vi "Read Message.vi"(8 "error in (no error)":errorcluster, 9 "timeout (0)":i32, 11 "Master CR in":refnum<class "Master CR.lvclass">) -> (0 "error out":errorcluster, 1 "timed out?":bool, 3 "Master CR out":refnum<class "Master CR.lvclass">)   [LabVIEW 2021, in "Master CR.lvclass"]
uses:
  Master CR.lvclass
  Master CR.lvclass/Master CR.ctl
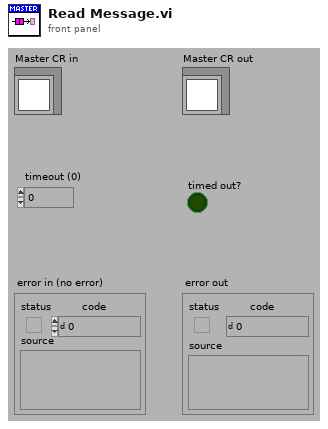
[diagram p1: front panel]
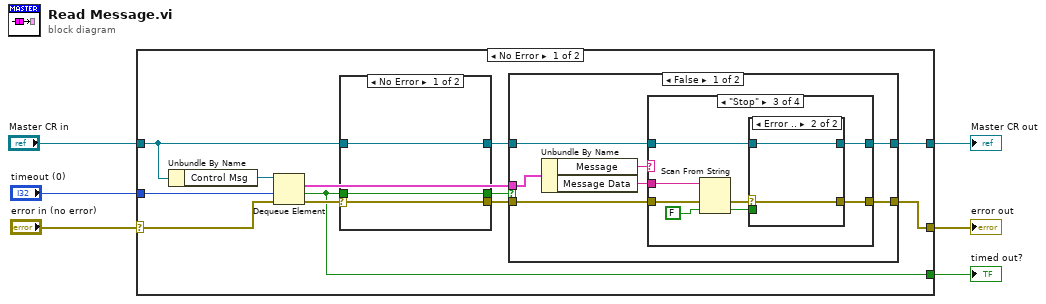
[diagram p0: block diagram]
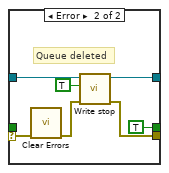
[diagram p2: hidden frame]
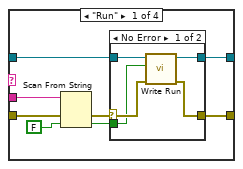
[diagram p3: hidden frame]
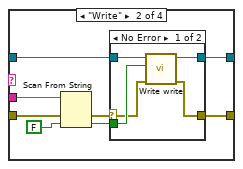
[diagram p5: hidden frame]
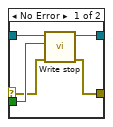
[diagram p7: hidden frame]
diagram:
  n1 = case shown="No Error" "error in (no error)" {
    selector: "error in (no error)" -> [w17 w86]
    tunnel: [w13 w86] -> w6
    tunnel: "timeout (0)" -> [w18 _]
    tunnel: [w14 w85] -> w1
    tunnel: [w10 _] -> w3
    tunnel: "Master CR in" -> [w8 w85]
    frame No Error {
      n2 = Unbundle By Name(w8) -> ("Control Msg"=w16:refnum<queue>)
      n3 = Dequeue Element(queue=w16, timeout in ms (-1)=w18, error in (no error)=w17) -> (element=w15:cluster{"Message":string, "Message Data":string}, timed out?=w10:bool, error out=w12:errorcluster)  [unwired: 1 out]
      n4 = case shown="No Error" w12 {
        selector: w12 -> [w21 w28]
        tunnel: [w21 w26] -> w11
        tunnel: w10 -> [w20 _]
        tunnel: [w20 TRUE ("timed out?")] -> w9
        tunnel: w8 -> [w19 w25]
        tunnel: [w19 w23] -> w7
        frame No Error {
        }
        frame Error {
          # "Queue deleted"
          n5 = call <vilib>:"Clear Errors.vi"("error in (no error)"=w28) -> ("error out"=w27:errorcluster)  [unwired: 5 in, 1 out]
          n6 = call "Write stop.vi"("error in (no error)"=w27, "Stop"=TRUE, "Master CR in"=w25) -> ("error out"=w26:errorcluster, "Master CR out"=w23:refnum<class "Master CR.lvclass">)  [unwired: 7 in]
        }
      }
      n7 = case shown="False" w9 {
        tunnel: w15 -> [w35 _]
        tunnel: w7 -> [w33 w84]
        tunnel: [w29 w84] -> w14
        tunnel: w11 -> [w31 w83]
        tunnel: [w30 w83] -> w13
        frame False {
          n8 = Unbundle By Name(w35) -> ("Message"=w34:string, "Message Data"=w32:string)
          n9 = case shown="\"Stop\"" w34 {
            tunnel: w33 -> [w38 w53 w68 w82]
            tunnel: w32 -> [w41 w56 w71 _]
            tunnel: [w43 w58 w73 w82] -> w29
            tunnel: w31 -> [w37 w52 w67 w81]
            tunnel: [w36 w51 w66 w81] -> w30
            frame "Run" {
              n10 = Scan From String(input string=w41, error in=w37, default 1=FALSE ("use system decimal point (T)")) -> (error out=w39:errorcluster, output 1=w40:bool)  [unwired: 2 in, 2 out]
              n11 = case shown="No Error" w39 {
                selector: w39 -> [w46 w49]
                tunnel: w38 -> [w48 w50]
                tunnel: [w47 w50] -> w43
                tunnel: w40 -> [w45 _]
                tunnel: [w44 w49] -> w36
                frame No Error {
                  n12 = call "Write Run.vi"("error in (no error)"=w46, "Run"=w45, "Master CR in"=w48) -> ("error out"=w44:errorcluster, "Master CR out"=w47:refnum<class "Master CR.lvclass">)  [unwired: 7 in]
                }
                frame Error {
                }
              }
            }
            frame "Write" {
              n13 = Scan From String(input string=w56, error in=w52, default 1=FALSE ("use system decimal point (T)")) -> (error out=w54:errorcluster, output 1=w55:bool)  [unwired: 2 in, 2 out]
              n14 = case shown="No Error" w54 {
                selector: w54 -> [w60 w64]
                tunnel: w53 -> [w63 w65]
                tunnel: [w62 w65] -> w58
                tunnel: w55 -> [w61 _]
                tunnel: [w59 w64] -> w51
                frame No Error {
                  n15 = call "Write write.vi"("error in (no error)"=w60, "Write"=w61, "Master CR in"=w63) -> ("error out"=w59:errorcluster, "Master CR out"=w62:refnum<class "Master CR.lvclass">)  [unwired: 7 in]
                }
                frame Error {
                }
              }
            }
            frame "Stop" {
              n16 = Scan From String(input string=w71, error in=w67, default 1=FALSE ("use system decimal point (T)")) -> (error out=w69:errorcluster, output 1=w70:bool)  [unwired: 2 in, 2 out]
              n17 = case shown="Error .." w69 {
                selector: w69 -> [w75 w79]
                tunnel: w68 -> [w77 w80]
                tunnel: [w78 w80] -> w73
                tunnel: w70 -> [w76 _]
                tunnel: [w74 w79] -> w66
                frame No Error {
                  n18 = call "Write stop.vi"("error in (no error)"=w75, "Stop"=w76, "Master CR in"=w77) -> ("error out"=w74:errorcluster, "Master CR out"=w78:refnum<class "Master CR.lvclass">)  [unwired: 7 in]
                }
                frame Error {
                }
              }
            }
            frame Default {
            }
          }
        }
        frame True {
        }
      }
    }
    frame Error {
    }
  }
  "error out" <- w6
  "timed out?" <- w3
  "Master CR out" <- w1
